vi "RunVis.vi"(6 "Re-Init":bool, 7 "Index":i8, 8 "dt":i8, 9 "HMI to Control":T1, 10 "SensorInputData":T2, 11 "arguments":string[](array[string])) -> (1 "Done":bool, 2 "HMI to Control Out":T1, 3 "SensorInputDataOut":T2)   [LabVIEW 2015]
uses:
  Typedefs/HMI_to_Control.ctl
  Typedefs/SensorInputData.ctl
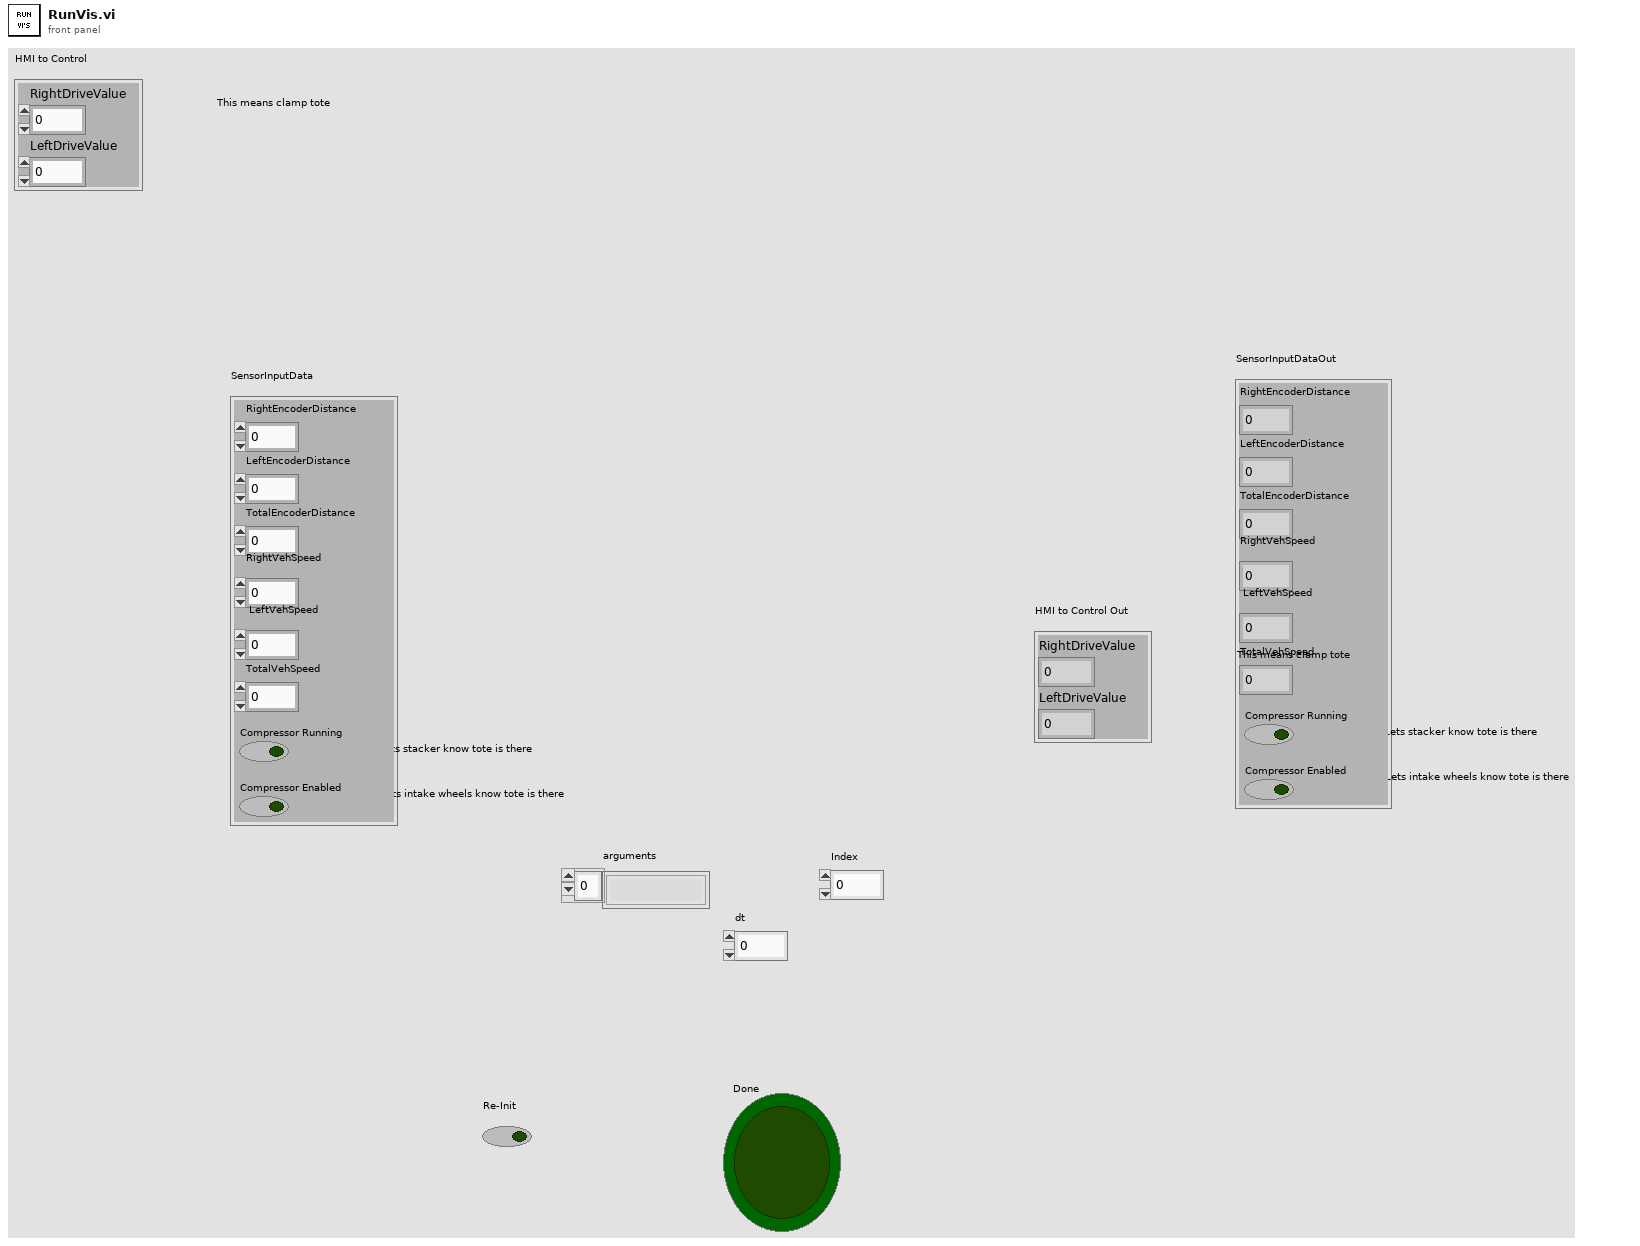
[diagram p1: front panel]
types:
  T1 = typedef "HMI_to_Control.ctl" = cluster{"RightDriveValue":dbl, "LeftDriveValue":dbl}
  T2 = typedef "SensorInputData.ctl" = cluster{"RightEncoderDistance":dbl, "LeftEncoderDistance":dbl, "TotalEncoderDistance":dbl, "RightVehSpeed":dbl, "LeftVehSpeed":dbl, "TotalVehSpeed":dbl, "Compressor Running":bool, "Compressor Enabled":bool}
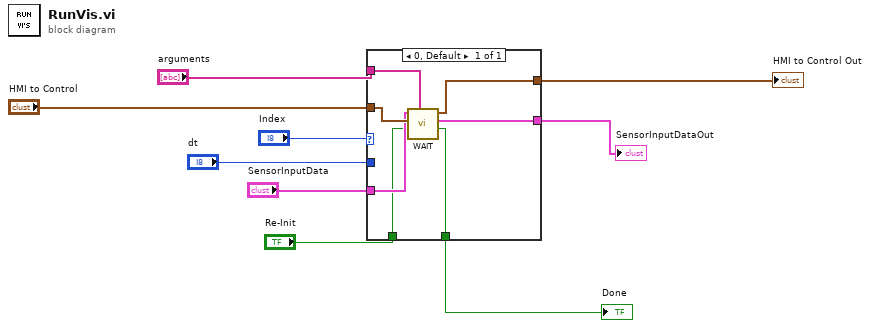
[diagram p0: block diagram]
diagram:
  n1 = case shown="0, Default" "Index" {
    tunnel: "HMI to Control" -> [w15]
    tunnel: "SensorInputData" -> [w14]
    tunnel: "Re-Init" -> [w13]
    tunnel: "arguments" -> [w16]
    tunnel: "dt" -> [_]
    tunnel: [w12] -> w3
    tunnel: [w11] -> w2
    tunnel: [w10] -> w1
    frame 0, Default {
      n2 = call "WAIT.vi"("arguments"=w16, "Reinit"=w13, "HMI to Control"=w15, "SensorInputData"=w14) -> ("Done"=w12:bool, "SensorInputDataOut"=w10:T2, "HMI to Control Out"=w11:T1)  [unwired: 5 in]
    }
  }
  "SensorInputDataOut" <- w1
  "HMI to Control Out" <- w2
  "Done" <- w3
